vi "Station Detail Main.vi"(8 "error in (no error)":errorcluster, 11 "LaserDetect01 in":refnum<class "LaserDetect01.lvclass">) -> (0 "error out":errorcluster, 2 "Station Out":T1=enum."ImformOut", 3 "LaserDetect01 out":refnum<class "LaserDetect01.lvclass">)   [LabVIEW 2019, in "LaserDetect01.lvclass"]
uses:
  LaserDetect01.lvclass
  Ctrl/Station Action.ctl
  BarcodeScan/Ctl/BarcodeStep.ctl
  Ctl/Laser Act Step.ctl
  Ctl/S11 PC to PLC.ctl
  Ctrl/Auto Inspection Station Name2.ctl
  Ctrl/Auto Inspection Data Name.ctl
  Ctl/S11 Station IO.ctl
  Ctrl/ModbusCmd.ctl
  Ctrl/MeasureDisplayTab.ctl
  Ctrl/Table Save.ctl
  Global/Process Global.vi
  LLB/Commonly VI/Main Glb.vi
  LLB/Commonly VI.lvlib
panel:
  out "Laser Point Data2":string
  out "Laser Point Data1":string
  in  "站別":i32
  out "Laser Data Read2":dbl
  out "Laser Data Read1":dbl
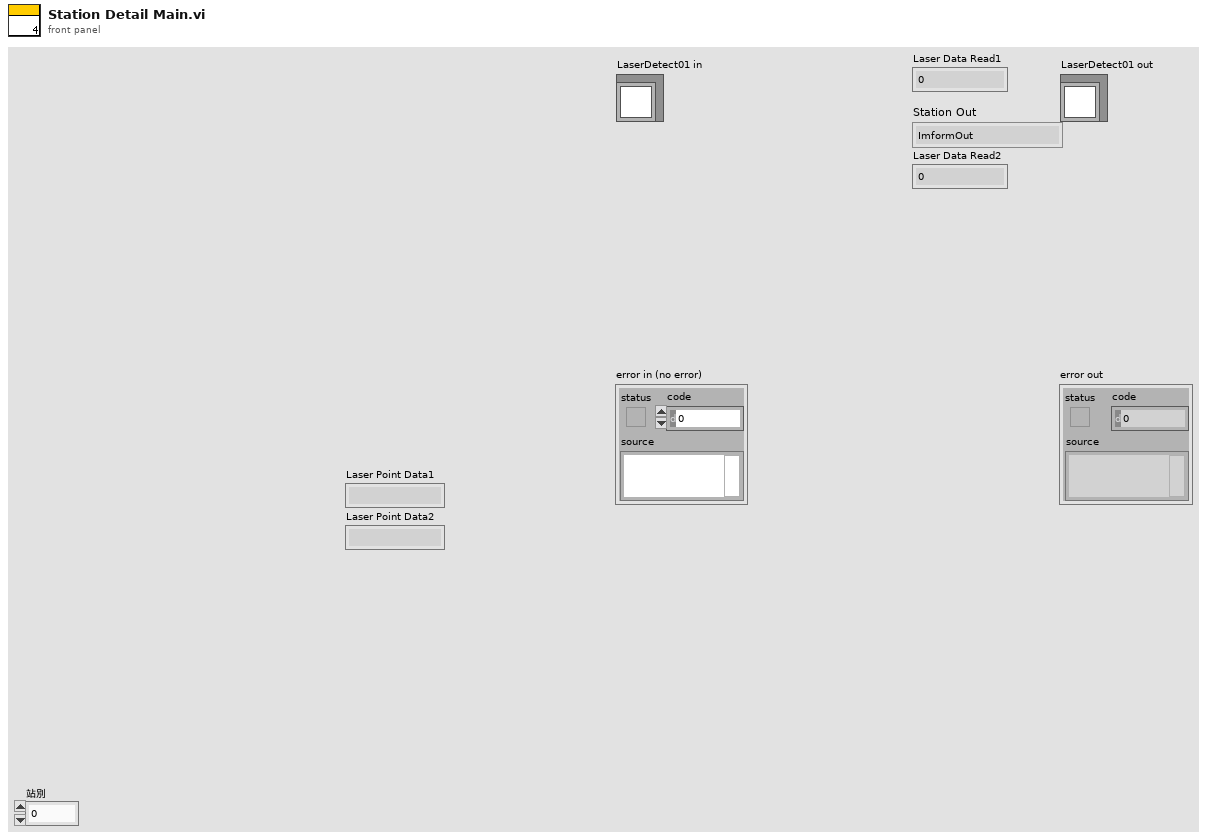
[diagram p1: front panel]
types:
  T1 = typedef "Station Action.ctl" = enum16{"Wait Item In", "Dectect Action", "ImformOut"}
  T2 = typedef "BarcodeStep.ctl" = enum16{"Initial", "BarcodeScan", "BcdCheck", "BcdCheckOK", "ReadPLCBarcode", "BcdCheckNG", "Merge", "SendPLC_OK", "DataSave", "IOSignal Off", "Finish"}
  T3 = typedef "S11 PC to PLC.ctl" = enum16{"S11雷射測高載盤有料", "雷射測量點1可測訊號", "雷射測量點2可測訊號"}
  T4 = typedef "Auto Inspection Data Name.ctl" = enum16{"LocalRun", "ItemSN(TimeCode)", "CurrentAction", "Error", "Data", "OKNG", "電壓值", "電壓值判斷", "電流值", "電流值判斷", "Laser1 Data", "Laser2 Data", "Laser OKNG", "StationNO"}
  T5 = typedef "Auto Inspection Station Name2.ctl" = enum16{"S1Barcode", "S2Measure", "S3Measure", "S4Measure", "S5Measure", "S11_LaserCheck", "S8_Vision AI"}
  T6 = cluster{"starting address":u16, "number of inputs":u16, "Sat Coils":bool[], "Holding Registers":u16[]}
  T7 = typedef "ModbusCmd.ctl" = enum16{"Connect", "Disconnect", "Init", "Fetch Basic Objects", "Fetch Input Refisters", "Fetch Discrete Inputs", "Set Coils", "Set Holding Registers", "Write Single Holding", "Exit"}
  T8 = typedef "Laser Act Step.ctl" = enum16{"Initial", "LaserCheck1", "Laser1Finish", "LaserCheck2", "Laser2Finish", "DataCheck", "NGWay", "OKWay", "DataSave", "Finish"}
  T9 = typedef "MeasureDisplayTab.ctl" = enum16{"Tray Barcode", "PCBA BARCODE", "硬體(Tool初始化)", "company(Tool初始化)", "耗電流 uA(電流表)", "電池負載電壓", "晶片ID(Tool FORMAT)", "雷雕ID(TOOl scan、藍芽接收器)", "Format(Tool FORMAT)", "Programe(Tool Programe)", "MAC(藍芽接收器)", "ID(藍芽接收器)", "KPA(藍芽接收器)", "溫度(藍芽接收器)", "SENSOR電池電壓(藍芽接收器)", "RSSI(藍芽接收器)", "SensorType_315(FSK scan)", "FSKsnVol_315(FSK scan)", "FSKscanl_315(FSK scan)", "P_315(FSK scan)", "T_315(FSK scan)", "SensorType_433(ASK scan)", "ASKsnVol_433(ASK scan)", "ASKscan_433(ASK scan)", "P_433(ASK scan)", "T_433(ASK scan)", "測高Data"}
  T10 = typedef "Table Save.ctl" = enum16{"initial", "Add", "Write", "Replace", "Delete", "REad", "RedTable", "Load"}
  T11 = typedef "S11 Station IO.ctl" = enum16{"S11雷射測量動作中", "S11雷射測點1完成", "S11雷射測點2完成", "S11雷測測量OK", "S11雷測測量NG", "S11雷測測量重測", "S11備用_6", "S11備用_7", "S11備用_8", "S11雷射測高完成"}
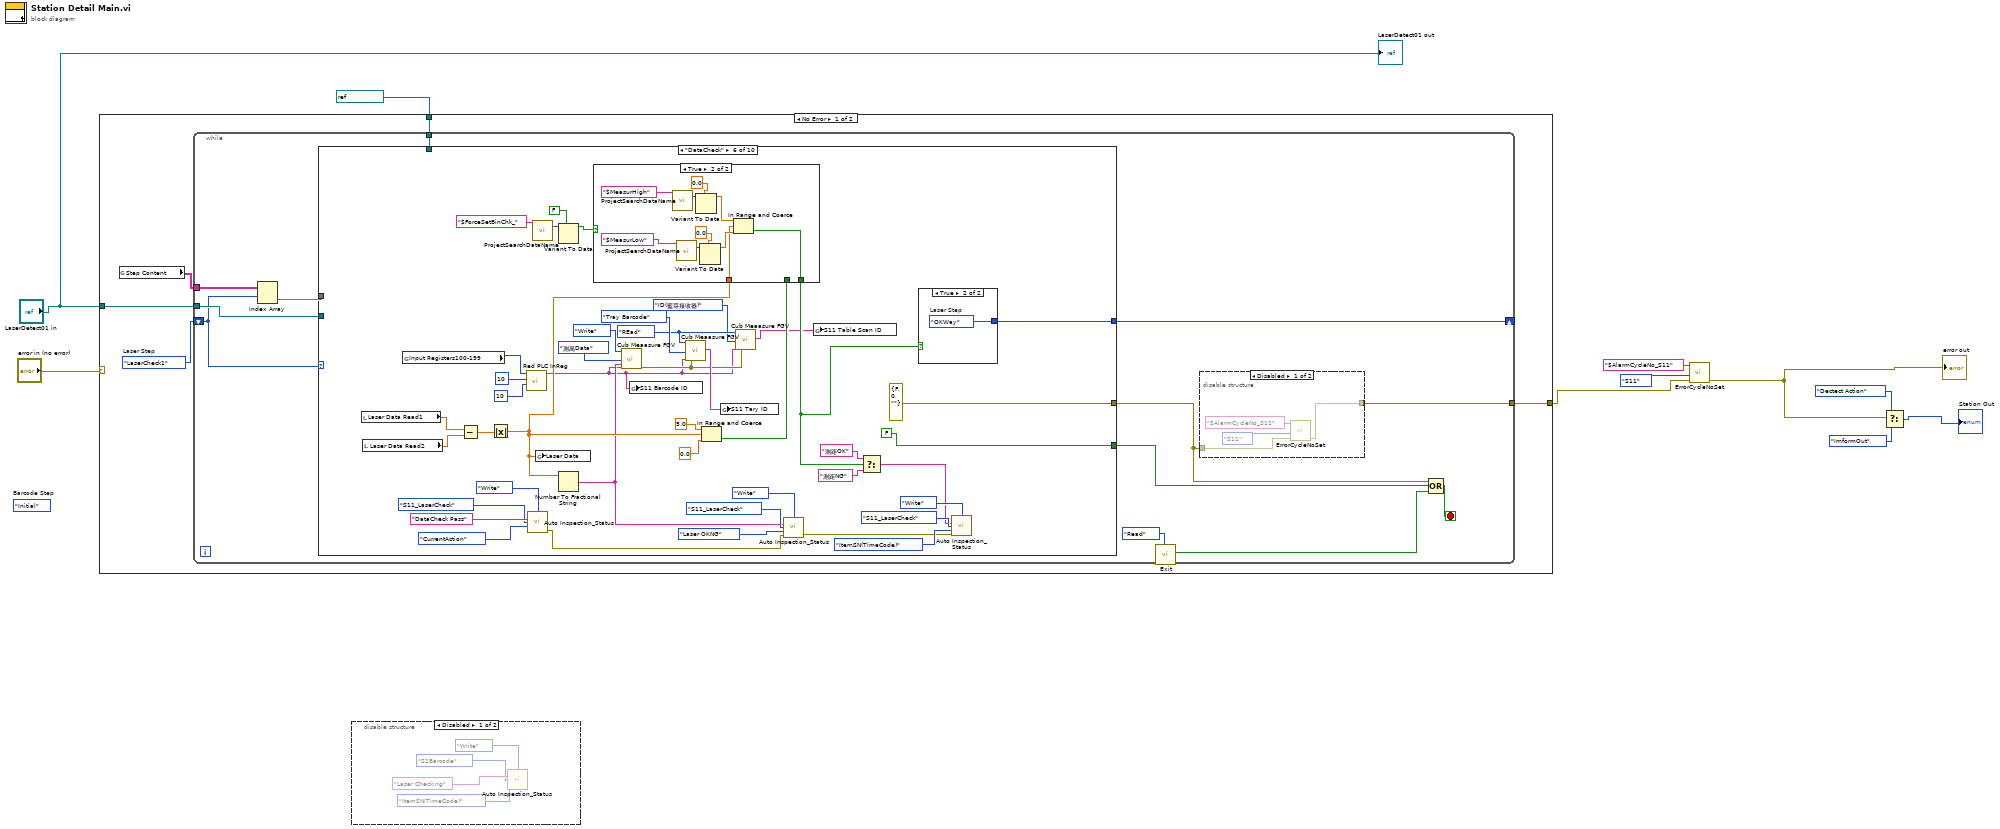
[diagram p0: block diagram]
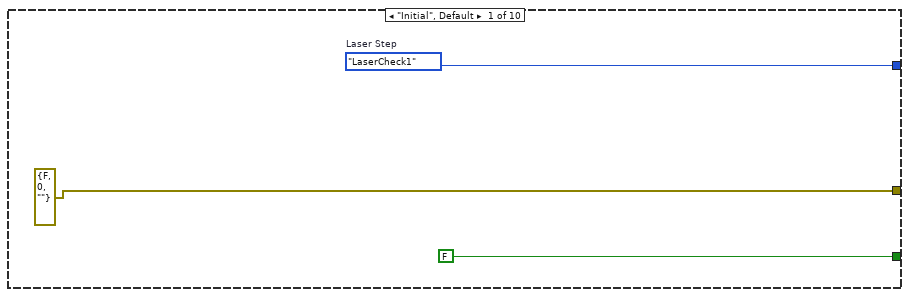
[diagram p4: hidden frame]
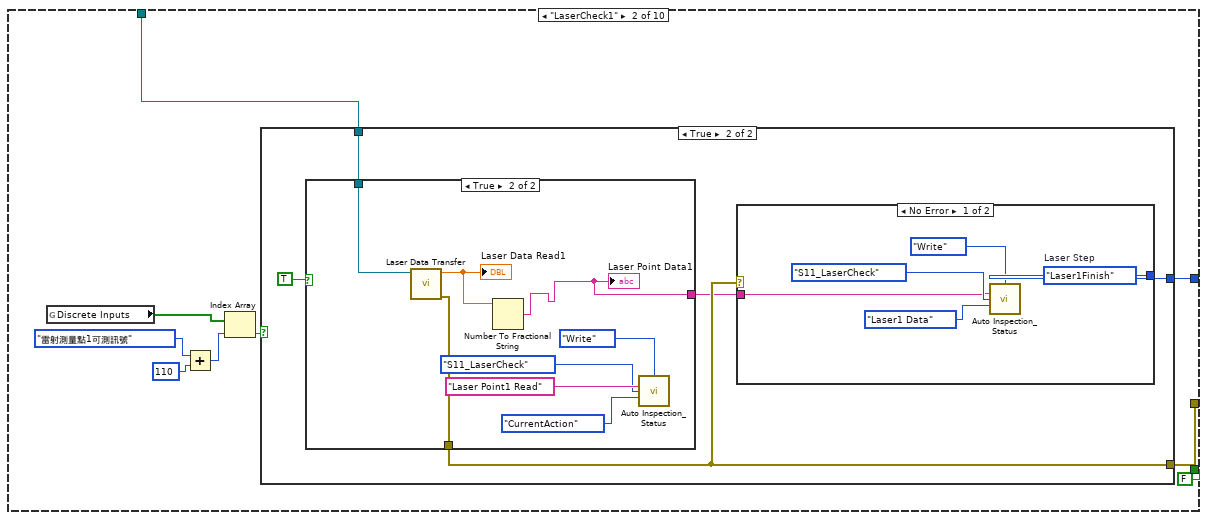
[diagram p5: hidden frame]
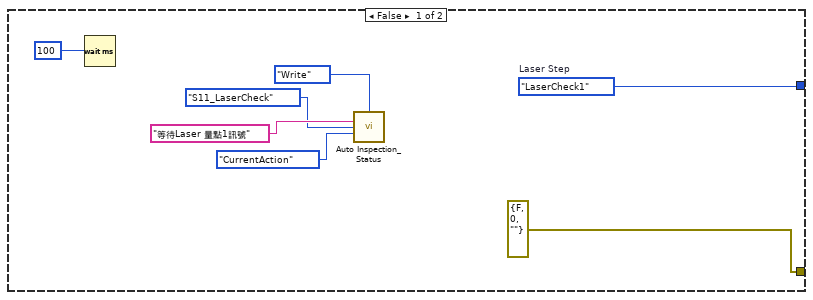
[diagram p6: hidden frame]
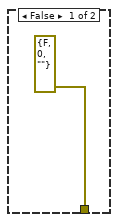
[diagram p7: hidden frame]
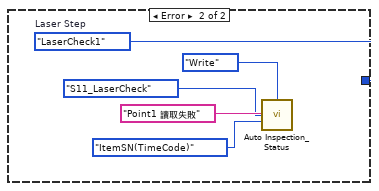
[diagram p8: hidden frame]
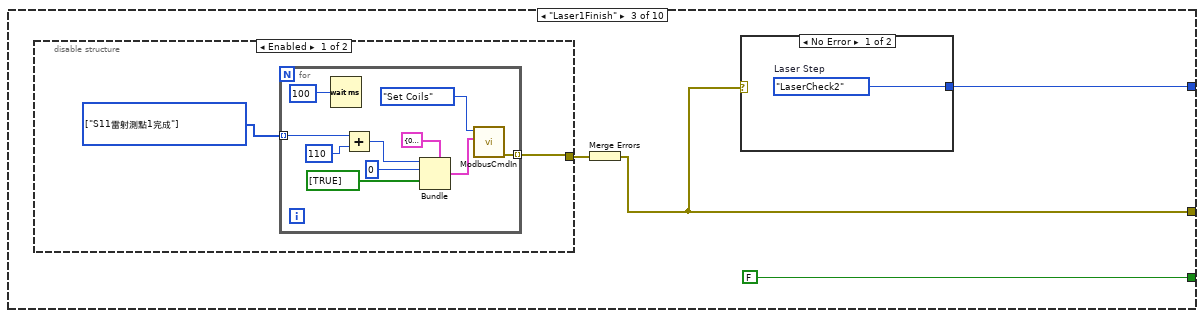
[diagram p9: hidden frame]
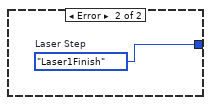
[diagram p10: hidden frame]
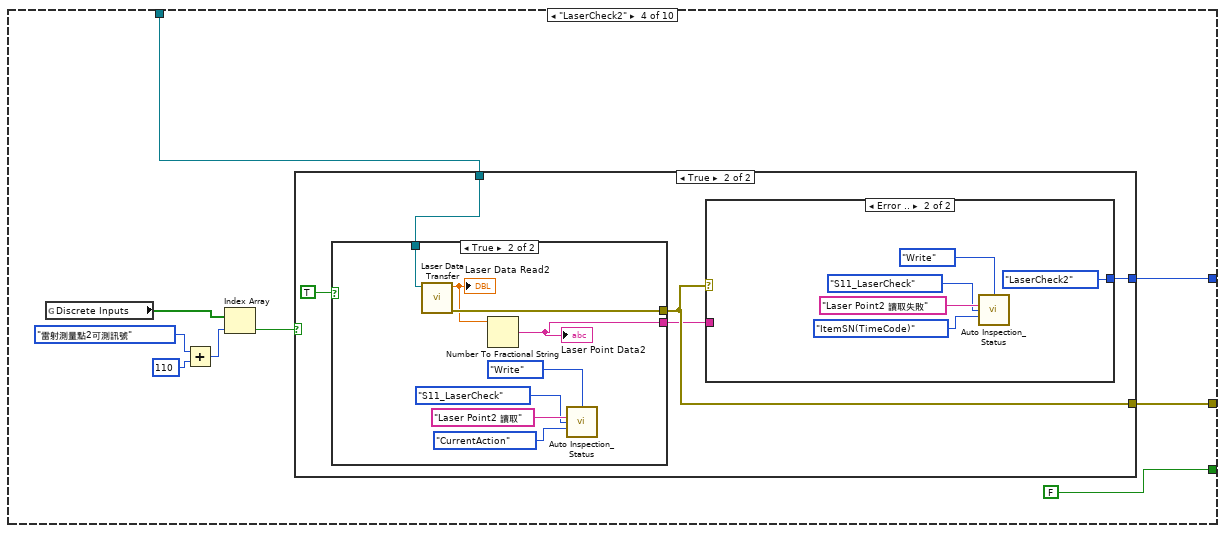
[diagram p12: hidden frame]
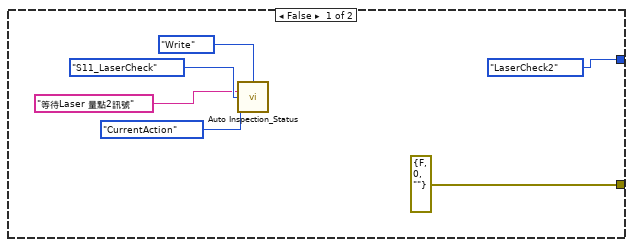
[diagram p13: hidden frame]
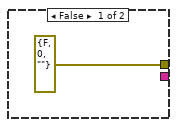
[diagram p14: hidden frame]
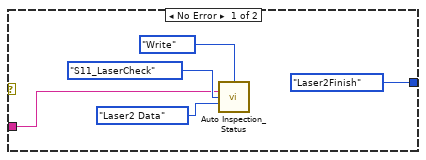
[diagram p15: hidden frame]
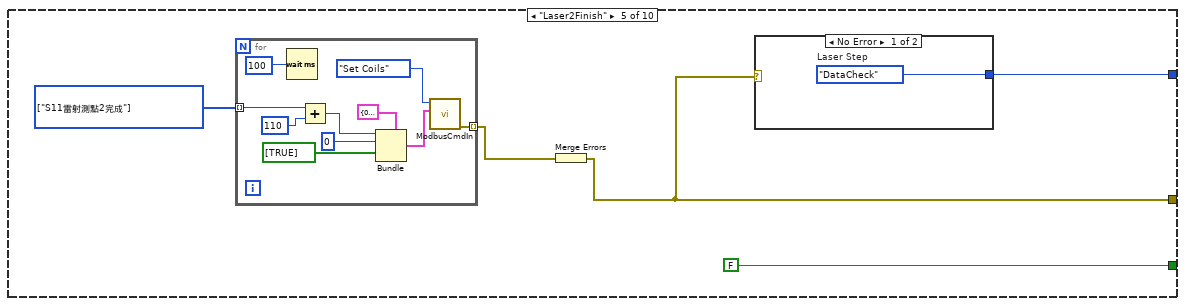
[diagram p16: hidden frame]
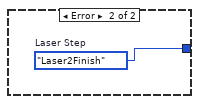
[diagram p17: hidden frame]
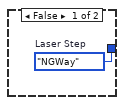
[diagram p18: hidden frame]
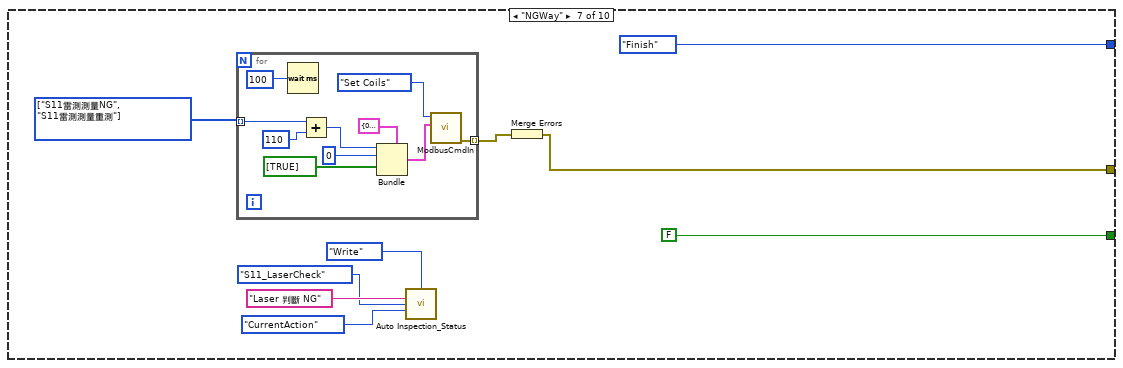
[diagram p20: hidden frame]
diagram:
  (unwired) BarcodeStep."Initial"  # Barcode Step
  n1 = case shown="No Error" "error in (no error)" {
    selector: "error in (no error)" -> [_ w250]
    tunnel: [w15 w250] -> w2
    tunnel: "LaserDetect01 in" -> [w14 _]
    tunnel: refnum<visa-resource-name> "COM13" ("VISA resource name") -> [w11 _]
    frame No Error {
      w12 = Laser_Act_Step."LaserCheck1"  # Laser Step
      n2 = global read "Process Global.vi" "Step Content"() -> (w13:string[][])
      n3 = while {
        tunnel: [w16] -> w15
        shift-right: [w27] -> _
        shift-left: w12 -> [w23]
        tunnel: w14 -> [w24]
        tunnel: w13 -> [w25]
        tunnel: w11 -> [w20]
        stop <- w22 stop-if-true
        n4 = Index Array(array=w25, index (row)=w23) -> (element=w26:string[])  [unwired: 1 in]
        n5 = case shown="\"DataCheck\"" w23 {
          tunnel: [errorcluster {"status"=FALSE, "code"=0, "source"=""} ("error constant") w42 w76 w102 w133 errorcluster {"status"=FALSE, "code"=0, "source"=""} ("error IO") w210 w229 errorcluster {"status"=FALSE, "code"=0, "source"=""} ("error IO") errorcluster {"status"=FALSE, "code"=0, "source"=""} ("error IO")] -> w17
          tunnel: [w33 w44 w78 w101 w136 w192 Laser_Act_Step."Finish" ("Laser Step") w233 w246 w249] -> w27
          tunnel: w24 -> [_ _ _ _ _ _ _ _ _ _]
          tunnel: w26 -> [_ _ _ _ _ _ _ _ _ _]
          tunnel: [FALSE FALSE FALSE FALSE FALSE FALSE FALSE FALSE FALSE TRUE] -> w21
          tunnel: w20 -> [_ w41 _ w100 _ _ _ _ _ _]
          frame "Initial", Default {
            w33 = Laser_Act_Step."LaserCheck1"  # Laser Step
          }
          frame "LaserCheck1" {
            n6 = global read "Main Glb.vi" "Discrete Inputs"() -> (w40:bool[])
            n7 = Add(x=S11_PC_to_PLC."雷射測量點1可測訊號", y=110) -> (x+y=w39:i32)
            n8 = Index Array(array=w40, index=w39) -> (element=w36:bool)
            n9 = case shown="True" w36 {
              tunnel: [w51 w56] -> w44
              tunnel: [errorcluster {"status"=FALSE, "code"=0, "source"=""} ("error out") w55] -> w42
              tunnel: w41 -> [_ w53]
              frame False {
                w51 = Laser_Act_Step."LaserCheck1"  # Laser Step
                n10 = Wait (ms)(milliseconds to wait=100) -> ()  [unwired: 1 out]
                n11 = call "Auto Inspection_Status.vi"("Action"=enum16{"Initial", "Write", "Read"}."Write", "DataIn"="等待Laser 量點1訊號", "Station"=Auto_Inspection_Station_Name2."S11_LaserCheck", "Data"=Auto_Inspection_Data_Name."CurrentAction") -> ()  [unwired: 9 in, 3 out]
              }
              frame True {
                n12 = case shown="True" TRUE {
                  tunnel: [errorcluster {"status"=FALSE, "code"=0, "source"=""} ("error out") w65] -> w55
                  tunnel: w53 -> [_ w63]
                  tunnel: [_ w62] -> w52
                  frame False {
                  }
                  frame True {
                    n13 = call "Laser Data Transfer.vi"("VISA resource name"=w63) -> ("error out"=w65:errorcluster, "Laser Data Read"=w64:dbl)  [unwired: 9 in]
                    "Laser Data Read1" <- w64
                    n14 = Number To Fractional String(number=w64) -> (F-format string=w62:string)  [unwired: 3 in]
                    "Laser Point Data1" <- w62
                    n15 = call "Auto Inspection_Status.vi"("Action"=enum16{"Initial", "Write", "Read"}."Write", "DataIn"="Laser Point1 Read", "Station"=Auto_Inspection_Station_Name2."S11_LaserCheck", "Data"=Auto_Inspection_Data_Name."CurrentAction") -> ()  [unwired: 9 in, 3 out]
                  }
                }
                n16 = case shown="No Error" w55 {
                  tunnel: [w70 w75] -> w56
                  tunnel: w52 -> [w66 _]
                  frame No Error {
                    w70 = Laser_Act_Step."Laser1Finish"  # Laser Step
                    n17 = call "Auto Inspection_Status.vi"("Action"=enum16{"Initial", "Write", "Read"}."Write", "DataIn"=w66, "Station"=Auto_Inspection_Station_Name2."S11_LaserCheck", "Data"=Auto_Inspection_Data_Name."Laser1 Data") -> ()  [unwired: 9 in, 3 out]
                  }
                  frame Error {
                    w75 = Laser_Act_Step."LaserCheck1"  # Laser Step
                    n18 = call "Auto Inspection_Status.vi"("Action"=enum16{"Initial", "Write", "Read"}."Write", "DataIn"="Point1 讀取失敗", "Station"=Auto_Inspection_Station_Name2."S11_LaserCheck", "Data"=Auto_Inspection_Data_Name."ItemSN(TimeCode)") -> ()  [unwired: 9 in, 3 out]
                  }
                }
              }
            }
          }
          frame "Laser1Finish" {
            n19 = disable-structure shown="Enabled" {
              disable-tunnel: [w82 _] -> w79
              frame Enabled {
                w83 = T11[] [enum."S11雷射測點1完成"] items=["S11雷射測量動作中", "S11雷射測點1完成", "S11雷射測點2完成", "S11雷測測量OK", "S11雷測測量NG", "S11雷測測量重測", "S11備用_6", "S11備用_7", "S11備用_8", "S11雷射測高完成"]
                n20 = for {
                  tunnel: w83 -> [w86] mode=indexing
                  tunnel: [w84] -> w82 mode=indexing
                  n21 = Wait (ms)(milliseconds to wait=100) -> ()  [unwired: 1 out]
                  n22 = Add(x=w86, y=u16 110 ("starting address")) -> (x+y=w93:u16)
                  n23 = Bundle(cluster=T6 {"starting address"=0, "number of inputs"=0, "Sat Coils"=[], "Holding Registers"=[]} ("data"), "starting address"=w93, "number of inputs"=u16 0, "Sat Coils"=bool[] [TRUE]) -> (w88:T6)  [unwired: 1 in]
                  n24 = call "ModbusCmdIn.vi"("data"=w88, "Enum"=ModbusCmd."Set Coils") -> ("error out"=w84:errorcluster)  [unwired: 9 in]
                }
              }
              frame Disabled {
              }
            }
            n25 = Merge Errors(w79) -> (w76:errorcluster)
            n26 = case shown="No Error" w76 {
              tunnel: [w80 w81] -> w78
              frame No Error {
                w80 = Laser_Act_Step."LaserCheck2"  # Laser Step
              }
              frame Error {
                w81 = Laser_Act_Step."Laser1Finish"  # Laser Step
              }
            }
          }
          frame "LaserCheck2" {
            n27 = global read "Main Glb.vi" "Discrete Inputs"() -> (w99:bool[])
            n28 = Add(x=S11_PC_to_PLC."雷射測量點2可測訊號", y=110) -> (x+y=w96:i32)
            n29 = Index Array(array=w99, index=w96) -> (element=w95:bool)
            n30 = case shown="True" w95 {
              tunnel: [errorcluster {"status"=FALSE, "code"=0, "source"=""} ("error out") w113] -> w102
              tunnel: [Laser_Act_Step."LaserCheck2" ("Laser Step") w112] -> w101
              tunnel: w100 -> [_ w110]
              frame False {
                n31 = call "Auto Inspection_Status.vi"("Action"=enum16{"Initial", "Write", "Read"}."Write", "DataIn"="等待Laser 量點2訊號", "Station"=Auto_Inspection_Station_Name2."S11_LaserCheck", "Data"=Auto_Inspection_Data_Name."CurrentAction") -> ()  [unwired: 9 in, 3 out]
              }
              frame True {
                n32 = case shown="True" TRUE {
                  tunnel: [errorcluster {"status"=FALSE, "code"=0, "source"=""} ("error out") w122] -> w113
                  tunnel: w110 -> [_ w120]
                  tunnel: [_ w115] -> w109
                  frame False {
                  }
                  frame True {
                    n33 = call "Laser Data Transfer.vi"("VISA resource name"=w120) -> ("error out"=w122:errorcluster, "Laser Data Read"=w121:dbl)  [unwired: 9 in]
                    "Laser Data Read2" <- w121
                    n34 = Number To Fractional String(number=w121) -> (F-format string=w115:string)  [unwired: 3 in]
                    "Laser Point Data2" <- w115
                    n35 = call "Auto Inspection_Status.vi"("Action"=enum16{"Initial", "Write", "Read"}."Write", "DataIn"="Laser Point2 讀取", "Station"=Auto_Inspection_Station_Name2."S11_LaserCheck", "Data"=Auto_Inspection_Data_Name."CurrentAction") -> ()  [unwired: 9 in, 3 out]
                  }
                }
                n36 = case shown="Error .." w113 {
                  tunnel: [Laser_Act_Step."Laser2Finish" ("Laser Step") Laser_Act_Step."LaserCheck2" ("Laser Step")] -> w112
                  tunnel: w109 -> [w123 _]
                  frame No Error {
                    n37 = call "Auto Inspection_Status.vi"("Action"=enum16{"Initial", "Write", "Read"}."Write", "DataIn"=w123, "Station"=Auto_Inspection_Station_Name2."S11_LaserCheck", "Data"=Auto_Inspection_Data_Name."Laser2 Data") -> ()  [unwired: 9 in, 3 out]
                  }
                  frame Error {
                    n38 = call "Auto Inspection_Status.vi"("Action"=enum16{"Initial", "Write", "Read"}."Write", "DataIn"="Laser Point2 讀取失敗", "Station"=Auto_Inspection_Station_Name2."S11_LaserCheck", "Data"=Auto_Inspection_Data_Name."ItemSN(TimeCode)") -> ()  [unwired: 9 in, 3 out]
                  }
                }
              }
            }
          }
          frame "Laser2Finish" {
            w137 = T11[] [enum."S11雷射測點2完成"] items=["S11雷射測量動作中", "S11雷射測點1完成", "S11雷射測點2完成", "S11雷測測量OK", "S11雷測測量NG", "S11雷測測量重測", "S11備用_6", "S11備用_7", "S11備用_8", "S11雷射測高完成"]
            n39 = for {
              tunnel: w137 -> [w142] mode=indexing
              tunnel: [w140] -> w135 mode=indexing
              n40 = Wait (ms)(milliseconds to wait=100) -> ()  [unwired: 1 out]
              n41 = Add(x=w142, y=u16 110 ("starting address")) -> (x+y=w149:u16)
              n42 = Bundle(cluster=T6 {"starting address"=0, "number of inputs"=0, "Sat Coils"=[], "Holding Registers"=[]} ("data"), "starting address"=w149, "number of inputs"=u16 0, "Sat Coils"=bool[] [TRUE]) -> (w144:T6)  [unwired: 1 in]
              n43 = call "ModbusCmdIn.vi"("data"=w144, "Enum"=ModbusCmd."Set Coils") -> ("error out"=w140:errorcluster)  [unwired: 9 in]
            }
            n44 = Merge Errors(w135) -> (w133:errorcluster)
            n45 = case shown="No Error" w133 {
              tunnel: [w138 w139] -> w136
              frame No Error {
                w138 = Laser_Act_Step."DataCheck"  # Laser Step
              }
              frame Error {
                w139 = Laser_Act_Step."Laser2Finish"  # Laser Step
              }
            }
          }
          frame "DataCheck" {
            w154 = Table_Save."REad" ("Enum")
            n46 = local read "Laser Data Read1"() -> (w185:dbl)
            n47 = local read "Laser Data Read2"() -> (w184:dbl)
            n48 = global read "Main Glb.vi" "Input Registers100-199"() -> (w157:u16[])
            n49 = Subtract(x=w185, y=w184) -> (x-y=w183:dbl)
            n50 = Absolute Value(x=w183) -> (abs(x)=w163:dbl)
            n51 = call "Red PLC InReg.vi"("length"=10, "index"=10, "Input Registers Arr"=w157) -> ("Rad In Reg"=w152:string)  [unwired: 7 in, 1 out]
            n52 = call "Auto Inspection_Status.vi"("Action"=enum16{"Initial", "Write", "Read"}."Write", "DataIn"="DataCheck Pass", "Station"=Auto_Inspection_Station_Name2."S11_LaserCheck", "Data"=Auto_Inspection_Data_Name."CurrentAction") -> ("error out"=w173:errorcluster)  [unwired: 9 in, 2 out]
            n53 = call "ProjectSearchDataName.vi"("element"="$ForceSetBinChk_") -> ("variant"=w178:variant)  [unwired: 7 in, 3 out]
            n54 = global write "Process Global.vi" "Laser Data"(w163) -> ()
            n55 = Number To Fractional String(number=w163) -> (F-format string=w160:string)  [unwired: 3 in]
            n56 = Variant To Data(type=FALSE, Variant=w178) -> (data=w179:bool)  [unwired: 1 in, 1 out]
            n57 = call "Cub Meaasure FGV.vi"("Action"=Table_Save."Write" ("Enum"), "Save Index"=MeasureDisplayTab."測高Data", "DataIn"=w160, "SN"=w152) -> ("error out"=w153:errorcluster)  [unwired: 8 in, 7 out]
            n58 = global write "Main Glb.vi" "S11 Barcode ID"(w152) -> ()
            n59 = call "Cub Meaasure FGV.vi"("Action"=w154, "Save Index"=MeasureDisplayTab."Tray Barcode", "SN"=w152, "error in (no error)"=w153) -> ("Read Index Data"=w155:string)  [unwired: 8 in, 7 out]
            n60 = In Range and Coerce(upper limit=5.0, x=w163, lower limit=0.0 ("upper limit")) -> (In Range?=w164:bool)  [unwired: 1 out]
            n61 = case shown="True" w179 {
              tunnel: w163 -> [_ w199]
              tunnel: [w195 w198] -> w167
              tunnel: w164 -> [w195 _]
              frame False {
              }
              frame True {
                n62 = call "ProjectSearchDataName.vi"("element"="$MeasurHigh") -> ("variant"=w204:variant)  [unwired: 7 in, 3 out]
                n63 = call "ProjectSearchDataName.vi"("element"="$MeasurLow") -> ("variant"=w203:variant)  [unwired: 7 in, 3 out]
                n64 = Variant To Data(type=0.0, Variant=w204) -> (data=w201:dbl)  [unwired: 1 in, 1 out]
                n65 = Variant To Data(type=0.0, Variant=w203) -> (data=w200:dbl)  [unwired: 1 in, 1 out]
                n66 = In Range and Coerce(upper limit=w201, x=w199, lower limit=w200) -> (In Range?=w198:bool)  [unwired: 1 out]
              }
            }
            n67 = global write "Main Glb.vi" "S11 Tary ID"(w155) -> ()
            n68 = call "Cub Meaasure FGV.vi"("Action"=w154, "Save Index"=MeasureDisplayTab."ID(藍芽接收器)", "SN"=w152, "error in (no error)"=w153) -> ("Read Index Data"=w150:string)  [unwired: 8 in, 7 out]
            n69 = call "Auto Inspection_Status.vi"("Action"=enum16{"Initial", "Write", "Read"}."Write", "DataIn"=w160, "Station"=Auto_Inspection_Station_Name2."S11_LaserCheck", "Data"=Auto_Inspection_Data_Name."Laser OKNG", "error in"=w173) -> ("error out"=w169:errorcluster)  [unwired: 8 in, 2 out]
            n70 = global write "Main Glb.vi" "S11 Table Scan ID"(w150) -> ()
            n71 = Select(t="測距OK", s=w167, f="測距NG") -> (s? t:f=w168:string)
            n72 = case shown="True" w167 {
              tunnel: [w193 w194] -> w192
              frame False {
                w193 = Laser_Act_Step."NGWay"  # Laser Step
              }
              frame True {
                w194 = Laser_Act_Step."OKWay"  # Laser Step
              }
            }
            n73 = call "Auto Inspection_Status.vi"("Action"=enum16{"Initial", "Write", "Read"}."Write", "DataIn"=w168, "Station"=Auto_Inspection_Station_Name2."S11_LaserCheck", "Data"=Auto_Inspection_Data_Name."ItemSN(TimeCode)", "error in"=w169) -> ()  [unwired: 8 in, 3 out]
          }
          frame "NGWay" {
            w212 = T11[] [enum."S11雷測測量NG", enum."S11雷測測量重測"] items=["S11雷射測量動作中", "S11雷射測點1完成", "S11雷射測點2完成", "S11雷測測量OK", "S11雷測測量NG", "S11雷測測量重測", "S11備用_6", "S11備用_7", "S11備用_8", "S11雷射測高完成"]
            n74 = for {
              tunnel: w212 -> [w217] mode=indexing
              tunnel: [w215] -> w211 mode=indexing
              n75 = Wait (ms)(milliseconds to wait=100) -> ()  [unwired: 1 out]
              n76 = Add(x=w217, y=u16 110 ("starting address")) -> (x+y=w224:u16)
              n77 = Bundle(cluster=T6 {"starting address"=0, "number of inputs"=0, "Sat Coils"=[], "Holding Registers"=[]} ("data"), "starting address"=w224, "number of inputs"=u16 0, "Sat Coils"=bool[] [TRUE]) -> (w219:T6)  [unwired: 1 in]
              n78 = call "ModbusCmdIn.vi"("data"=w219, "Enum"=ModbusCmd."Set Coils") -> ("error out"=w215:errorcluster)  [unwired: 9 in]
            }
            n79 = call "Auto Inspection_Status.vi"("Action"=enum16{"Initial", "Write", "Read"}."Write", "DataIn"="Laser 判斷 NG", "Station"=Auto_Inspection_Station_Name2."S11_LaserCheck", "Data"=Auto_Inspection_Data_Name."CurrentAction") -> ()  [unwired: 9 in, 3 out]
            n80 = Merge Errors(w211) -> (w210:errorcluster)
          }
          frame "OKWay" {
            w230 = T11[] [enum."S11雷測測量OK"] items=["S11雷射測量動作中", "S11雷射測點1完成", "S11雷射測點2完成", "S11雷測測量OK", "S11雷測測量NG", "S11雷測測量重測", "S11備用_6", "S11備用_7", "S11備用_8", "S11雷射測高完成"]
            w233 = Laser_Act_Step."DataSave"  # Laser Step
            # "給PLC訊號"
            n81 = call "Auto Inspection_Status.vi"("Action"=enum16{"Initial", "Write", "Read"}."Write", "DataIn"="Laser 測距OK", "Station"=Auto_Inspection_Station_Name2."S11_LaserCheck", "Data"=Auto_Inspection_Data_Name."CurrentAction") -> ()  [unwired: 9 in, 3 out]
            n82 = for {
              tunnel: w230 -> [w236] mode=indexing
              tunnel: [w234] -> w231 mode=indexing
              n83 = Wait (ms)(milliseconds to wait=100) -> ()  [unwired: 1 out]
              n84 = Add(x=w236, y=u16 110 ("starting address")) -> (x+y=w243:u16)
              n85 = Bundle(cluster=T6 {"starting address"=0, "number of inputs"=0, "Sat Coils"=[], "Holding Registers"=[]} ("data"), "starting address"=w243, "number of inputs"=u16 0, "Sat Coils"=bool[] [TRUE]) -> (w238:T6)  [unwired: 1 in]
              n86 = call "ModbusCmdIn.vi"("data"=w238, "Enum"=ModbusCmd."Set Coils") -> ("error out"=w234:errorcluster)  [unwired: 9 in]
            }
            n87 = Merge Errors(w231) -> (w229:errorcluster)
          }
          frame "DataSave" {
            w246 = Laser_Act_Step."Finish"  # Laser Step
            n88 = disable-structure shown="Disabled" {
              frame Disabled {
                n89 = local read "Laser Data Read2"() -> ()  [unwired: 1 in]
                n90 = local read "Laser Data Read1"() -> ()  [unwired: 1 in]
                n91 = local read "Laser Point Data2"() -> ()  [unwired: 1 in]
              }
              frame Enabled {
              }
            }
          }
          frame "Finish" {
            w249 = Laser_Act_Step."Initial"  # Laser Step
          }
        }
        n92 = call "Exit.vi"("Enum"=enum16{"Initial", "Read", "Write"}."Read") -> ("ExitOut"=w18:bool)  [unwired: 10 in]
        n93 = disable-structure shown="Disabled" {
          disable-tunnel: w17 -> [w29 w32]
          disable-tunnel: [w28 w32] -> w16
          frame Disabled {
            n94 = call "ErrorCycleNoSet.vi"("error in"=w29, "CaseNo"=enum16{"S2", "S3", "S4", "S11"}."S11", "Error Set Item"="$AlarmCycleNo_S11") -> ("error out"=w28:errorcluster)  [unwired: 8 in]
          }
          frame Enabled {
          }
        }
        n95 = Compound Arithmetic op=OR(w17, w21, w18) -> (w22:bool)
      }
    }
    frame Error {
    }
  }
  n96 = disable-structure shown="Disabled" {
    frame Disabled {
      n97 = call "Auto Inspection_Status.vi"("Action"=enum16{"Initial", "Write", "Read"}."Write", "DataIn"="Laser Checking", "Station"=Auto_Inspection_Station_Name2."S1Barcode", "Data"=Auto_Inspection_Data_Name."ItemSN(TimeCode)") -> ()  [unwired: 9 in, 3 out]
    }
    frame Enabled {
    }
  }
  n98 = call "ErrorCycleNoSet.vi"("error in"=w2, "CaseNo"=enum16{"S2", "S3", "S4", "S11"}."S11", "Error Set Item"="$AlarmCycleNo_S11") -> ("error out"=w1:errorcluster)  [unwired: 8 in]
  "error out" <- w1
  n99 = Select(t=Station_Action."Dectect Action" ("Station Out"), s=w1, f=Station_Action."ImformOut" ("Station Out")) -> (s? t:f=→"Station Out":T1)
  "LaserDetect01 out" <- "LaserDetect01 in"
